vi "MoveArm.vi"() -> ()   [LabVIEW 2017]
panel:
  in  "Height":dbl
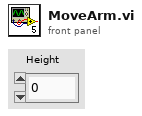
[diagram p1: front panel]
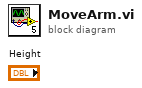
[diagram p0: block diagram]
diagram:
